vi "LinearSystemSim_ClampInput.vi"(9 "Battery_Volts":dbl, 11 "Input":T1) -> (0 "Size Coerced":bool, 3 "ClampedInput":T1)   [LabVIEW 2019, in "Trajectory_Library.lvlib"]
doc: "Clamp the input vector such that no element exceeds the given voltage. If any does, the relative magnitudes of the input will be maintained.\n \nInputs:\n - Input -- The input vector (u).\n - BatteryVolts -- The current battery voltage (volts)\n\nOutputs:\n - ClampedInput -- The normalized input.\n - SizeCoerced -- If TRUE, an error occured. Execution may continue."
uses:
  Trajectory_Library.lvlib
  <vilib>/Analysis/Matrix/Datatypes/RealMatrix.ctl
  <vilib>/Analysis/Matrix/NI_Matrix.lvlib
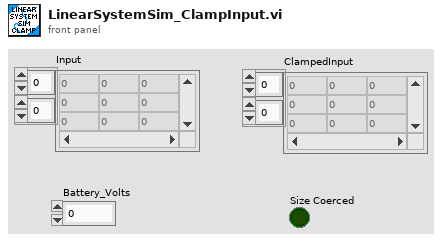
[diagram p1: front panel]
types:
  T1 = typedef "NI_Matrix.lvlib/RealMatrix.ctl" = dbl[][]
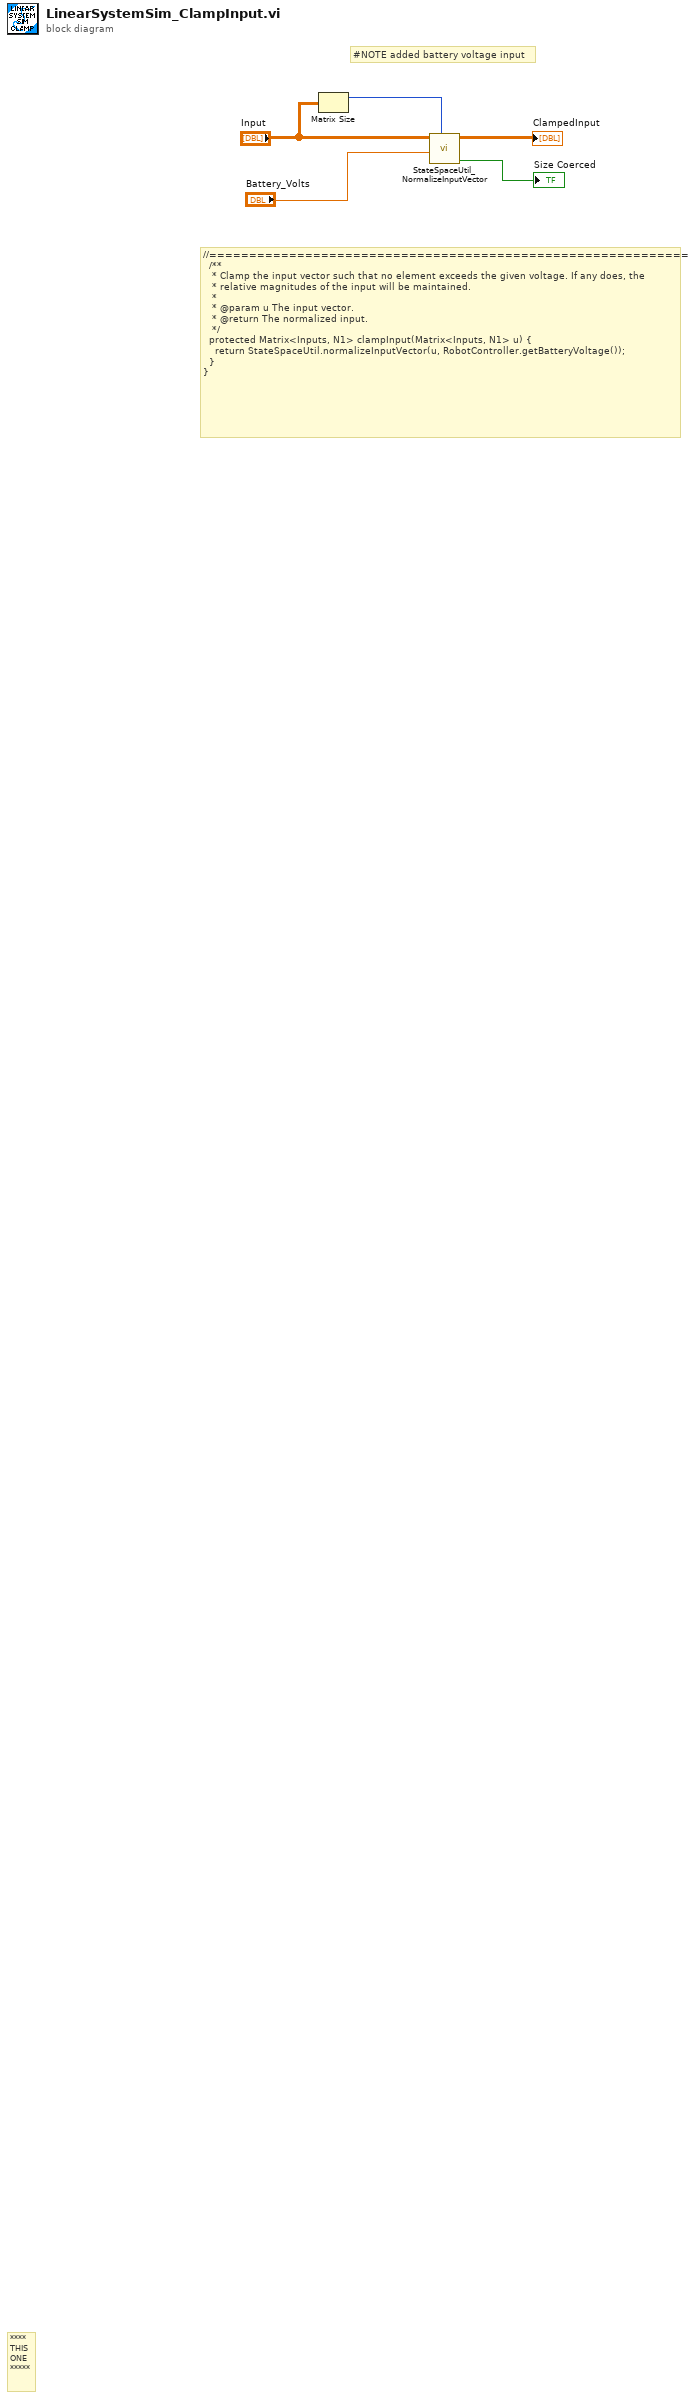
[diagram p0: block diagram]
diagram:
  # "#NOTE added battery voltage input"
  # "//============================================================\n  /**\n   * Clamp the input vector such that no element exceeds the given voltage. If any does, the\n   * relative magnitudes of the input will be maintained.\n   *\n   * @param u The input vector.\n   * @return The normalized input.\n   */\n  protected Matrix<Inputs, N1> clampInput(Matrix<Inputs, N1> u) {\n    return StateSpaceUtil.normalizeInputVector(u, RobotController.getBatteryVoltage());\n  }\n}"
  # "****\nTHIS\nONE\n*****"
  n1 = Matrix Size(0:"Input") -> (1:w3:i32)  [unwired: 1 out]
  n2 = call "StateSpaceUtil_NormalizeInputVector.vi"("J"=w3, "Max_Magnitude"="Battery_Volts", "U"="Input") -> ("Size Coerced"=→"Size Coerced":bool, "NormalizedU"=→"ClampedInput":T1)  [unwired: 7 in]
